vi "TSAPT-Post Log Message.vi"(8 "error in (no error)":errorcluster, 10 "LOG":string, 11 "Sequence Context In":refnum<k7>) -> (0 "error out":errorcluster)   [LabVIEW 2020]
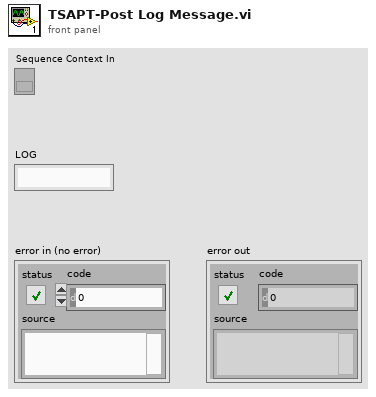
[diagram p1: front panel]
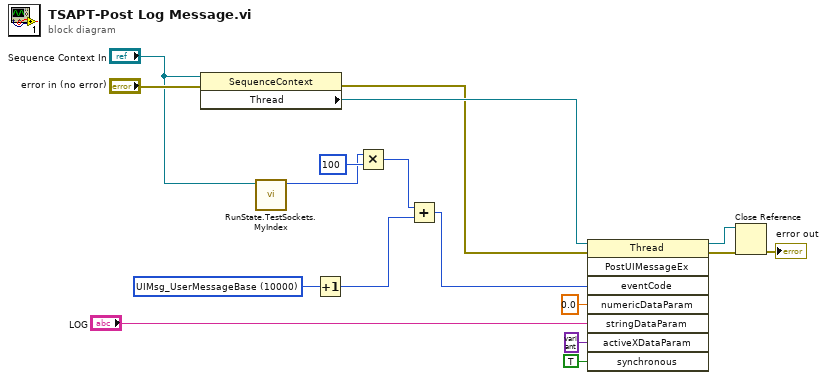
[diagram p0: block diagram]
diagram:
  w16 = 10000 items=["UIMsg_BreakOnUserRequest"=1, "UIMsg_BreakOnBreakpoint"=2, "UIMsg_BreakOnRunTimeError"=3, "UIMsg_Trace"=4, "UIMsg_TerminatingExecution"=5, "UIMsg_AbortingExecution"=6, "UIMsg_KillingExecutionThreads"=7, "UIMsg_EndExecution"=8, "UIMsg_ShutDownComplete"=9, "UIMsg_StartExecution"=10, "UIMsg_ProgressPercent"=11, "UIMsg_ProgressText"=12, "UIMsg_StartInteractiveExecution"=13, "UIMsg_EndInteractiveExecution"=14, "UIMsg_TerminatingInteractiveExecution"=15, "UIMsg_TerminationCancelled"=16, "UIMsg_ResumeFromBreak"=17, "UIMsg_StartFileExecution"=18, "UIMsg_EndFileExecution"=19, "UIMsg_ShutDownCancelled"=20, "UIMsg_LocalizationSettingChanged"=21, "UIMsg_OpenWindows"=22, "UIMsg_TileWindows"=23, "UIMsg_CascadeWindows"=24, "UIMsg_ReportChanged"=25, "UIMsg_CloseWindows"=26, "UIMsg_RefreshWindows"=27, "UIMsg_ClientFileChanged"=28, "UIMsg_DisplayReport"=29, "UIMsg_ModelState_Initializing"=30, "UIMsg_ModelState_Waiting"=31, "UIMsg_ModelState_Identified"=32, "UIMsg_ModelState_BeginTesting"=33, "UIMsg_ModelState_TestingComplete"=34, "UIMsg_ModelState_PostProcessingComplete"=35, "UIMsg_ModelState_EnabledStateSet"=36, "UIMsg_ReportLocationChanged"=37, "UIMsg_GotoLocation"=38, "UIMsg_PushUndoItem"=39, "UIMsg_OutputMessages"=40, "UIMsg_TypePaletteFileListChanged"=41, "UIMsg_NonTerminatableThreadsArePreventingTermination"=42, "UIMsg_ModelState_PostProcessing"=43, "UIMsg_ReportCollectionChanged"=44, "UIMsg_RuntimeError"=45, "UIMsg_UserMessageBase"=10000] ("eventCode")
  n1 = property class="SequenceContext"(reference="Sequence Context In", error in="error in (no error)") -> (error out=w13:errorcluster, "Thread"=w17:refnum<k7>)  [unwired: 1 out]
  n2 = call "RunState.TestSockets.MyIndex.vi"("Automation Refnum in"="Sequence Context In") -> ("Numeric"=w3:i32)  [unwired: 10 in]
  n3 = Increment(x=w16) -> (x+1=w2:i32)
  n4 = Multiply(x=w3, y=i64 100) -> (x*y=w4:i64)
  n5 = Add(x=w4, y=w2) -> (x+y=w1:i64)
  n6 = invoke class="Thread" method="PostUIMessageEx"(reference=w17, error in=w13, "eventCode"=w1, "numericDataParam"=0.0, "stringDataParam"="LOG", "activeXDataParam"=variant, "synchronous"=TRUE) -> (reference out=w14:refnum<k7>, error out=w15:errorcluster)  [unwired: 1 in, 6 out]
  n7 = Close Reference(reference=w14, error in (no error)=w15) -> (error out=→"error out":errorcluster)
